vi "Ophir SendFrequency.vi"(0 "Visa Session":refnum<visa-resource-name>, 1 "error in (no error)":errorcluster) -> (2 "dup Visa Session":refnum<visa-resource-name>, 3 "Value Number":dbl format="%.3e", 4 "Value String":string, 5 "error out":errorcluster)   [LabVIEW 2017]
doc: "SendFrequency.vi returns frequency measurement from instrument\nVersion 1.00\nLast Updated 16 March 2005\n\nInputs:\nVisa Session\nErrorIn\n\nOutputs:\ndup Visa Session\nValue Number is the measurement value\nValue String is the measurement string\nNote:\nIn case of Overrange Measure The string contains *OVER\nErrorOut\nReturns Error n# -1339 when Measurement Failed"
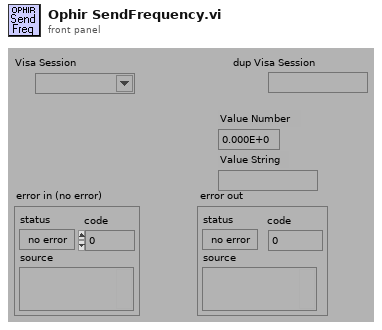
[diagram p1: front panel]
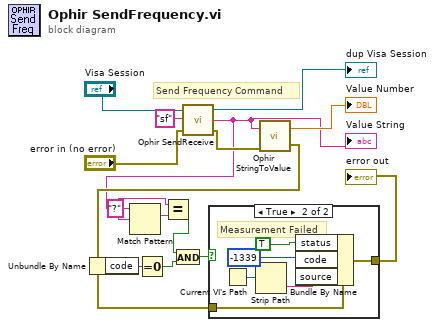
[diagram p0: block diagram]
diagram:
  w1 = "?"
  # "Send Frequency Command"
  n1 = call "Ophir SendReceive.vi"("error in (no error)"="error in (no error)", "Command"="sf", "Visa Session"="Visa Session") -> ("error out"=w11:errorcluster, "Frame Output"=w2:string, "dup Visa Session"=→"dup Visa Session":refnum<visa-resource-name>)
  "Value String" <- w2
  n2 = Match Pattern(string=w2, regular expression=w1) -> (match substring=w7:string)  [unwired: 4 out]
  n3 = Equal?(x=w1, y=w7) -> (x = y?=w6:bool)
  n4 = call "Ophir StringToValue.vi"("error in (no error)"=w11, "Frame"=w2) -> ("error out"=w4:errorcluster, "Value"=→"Value Number":dbl)
  n5 = Unbundle By Name(w4) -> ("code"=w9:i32)
  n6 = Equal To 0?(x=w9) -> (x = 0?=w8:bool)
  n7 = And(x=w6, y=w8) -> (x .and. y?=w5:bool)
  n8 = case shown="True" w5 {
    tunnel: w4 -> [w16 w19]
    tunnel: [w16 w18] -> w3
    frame False {
      # "No Error or \nError already exists"
    }
    frame True {
      # "Measurement Failed"
      n9 = Current VI's Path() -> (path=w17:path)
      n10 = Strip Path(path=w17) -> (name=w20:string)  [unwired: 1 out]
      n11 = Bundle By Name(cluster=w19, "status"=TRUE, "code"=-1339, "source"=w20) -> (w18:errorcluster)
    }
  }
  "error out" <- w3
